vi "MultiTool-Track-Generate-ndipolarisFileOutput-Q-vectors-Standalone.vi"() -> ()   [LabVIEW 2013]
panel:
  in  "File Identifier":string="Test"
  out "TIME":string
  out "Tool 2":T1={"Port Handle"="", "Frame Number"=0, "Tx"=0.0, "Ty"=0.0, "Tz"=0.0, "Q0"=0.0, "Qx"=0.0, "Qy"=0.0, "Qz"=0.0, "Deviation"=0.0, " Markers Missing"=TRUE, "Out of Volume"=TRUE} {"Deviation" format="%#.4f"; "Qz" format="%#.4f"; "Qy" format="%#.4f"; "Qx" format="%#.4f"; "Q0" format="%#.4f"; "Tz" format="%#.2f"; "Ty" format="%#.2f"; "Tx" format="%#.2f"}
  in  "Location of ROM File for Tool 2":path=path "C:/Program Files (x86)/Northern Digital Inc/8700339.rom"
  in  "NDI  Running":bool=TRUE
  out "Stop Reading":bool=TRUE
  out "Start Reading":bool
  in  "Track Outside Measurement Volume? (F:No)":bool
  in  "Track Stray Markers? (F:No)":bool
  out "Tool 1":T1={"Port Handle"="", "Frame Number"=0, "Tx"=0.0, "Ty"=0.0, "Tz"=0.0, "Q0"=0.0, "Qx"=0.0, "Qy"=0.0, "Qz"=0.0, "Deviation"=0.0, " Markers Missing"=TRUE, "Out of Volume"=TRUE} {"Deviation" format="%#.4f"; "Qz" format="%#.4f"; "Qy" format="%#.4f"; "Qx" format="%#.4f"; "Q0" format="%#.4f"; "Tz" format="%#.2f"; "Ty" format="%#.2f"; "Tx" format="%#.2f"}
  out "Measure loop":i32
  in  "Measuring":bool=TRUE
  in  "Output Directory":path=path "C:/Users/Diogo/Desktop/NDI-Labview Gripper"
  out "NDI Loop":i32
  in  "VISA resource name":refnum<visa-resource-name>="COM8"
  in  "Reset? (T:Yes)":bool=TRUE
  in  "Location of ROM File for Tool 1":path=path "C:/Program Files (x86)/Northern Digital Inc/8700449.rom"
  in  "Serial Configuration":T2={"Baud Rate (9600)"=9600, "Flow Control (0:None)"=0, "Parity"=0, "Data Bits"=8, "Stop Bits"=10} {"Stop Bits" items=["1.0"=10, "2.0"=20]; "Parity" items=["None", "Odd", "Even"]; "Flow Control (0:None)" items=["None", "XON/XOFF"]; "Baud Rate (9600)" items=["9600"=9600, "14.4k"=14400, "19.2k"=19200, "38.4k"=38400, "57.6k "=57600, "115.2k"=115200]}
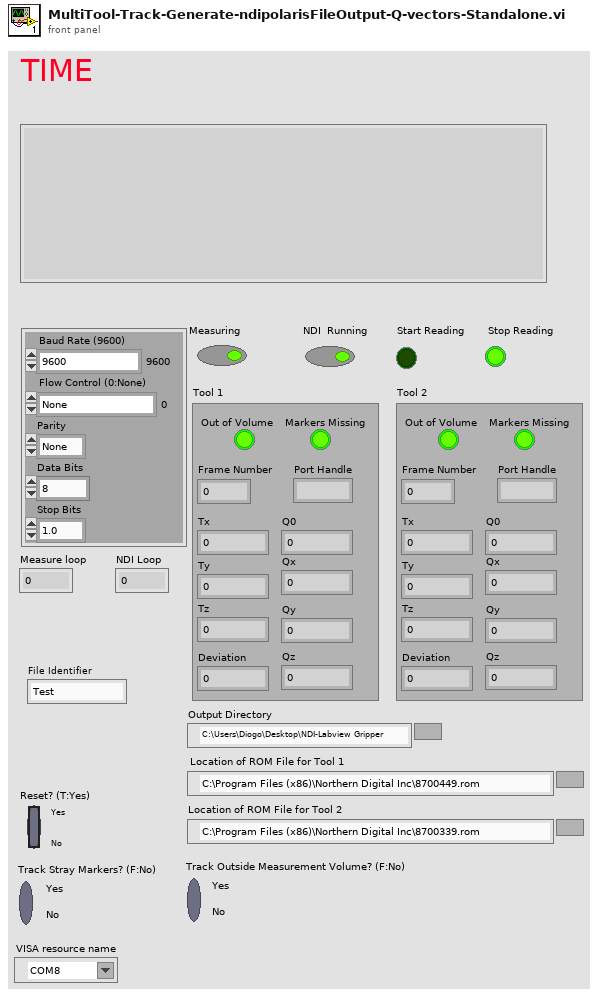
[diagram p1: front panel]
types:
  T1 = cluster{"Port Handle":string, "Frame Number":i32, "Tx":dbl, "Ty":dbl, "Tz":dbl, "Q0":dbl, "Qx":dbl, "Qy":dbl, "Qz":dbl, "Deviation":dbl, " Markers Missing":bool, "Out of Volume":bool}
  T2 = cluster{"Baud Rate (9600)":u32, "Flow Control (0:None)":u16, "Parity":u16, "Data Bits":u16, "Stop Bits":u16}
  T3 = cluster{"Port Handle":string, "Frame Number":u32, "Tx":dbl, "Ty":dbl, "Tz":dbl, "Q0":dbl, "Qx":dbl, "Qy":dbl, "Qz":dbl, "Deviation":dbl, "Missing?":bool, "Out of Volume?":bool}[]
  T4 = cluster{"Transformations[0]":cluster{"Port Handle":string, "Frame Number":u32, "Tx":dbl, "Ty":dbl, "Tz":dbl, "Q0":dbl, "Qx":dbl, "Qy":dbl, "Qz":dbl, "Deviation":dbl, "Missing?":bool, "Out of Volume?":bool}, "Transformations[1]":cluster{"Port Handle":string, "Frame Number":u32, "Tx":dbl, "Ty":dbl, "Tz":dbl, "Q0":dbl, "Qx":dbl, "Qy":dbl, "Qz":dbl, "Deviation":dbl, "Missing?":bool, "Out of Volume?":bool}, "Transformations[2]":cluster{"Port Handle":string, "Frame Number":u32, "Tx":dbl, "Ty":dbl, "Tz":dbl, "Q0":dbl, "Qx":dbl, "Qy":dbl, "Qz":dbl, "Deviation":dbl, "Missing?":bool, "Out of Volume?":bool}, "Transformations[3]":cluster{"Port Handle":string, "Frame Number":u32, "Tx":dbl, "Ty":dbl, "Tz":dbl, "Q0":dbl, "Qx":dbl, "Qy":dbl, "Qz":dbl, "Deviation":dbl, "Missing?":bool, "Out of Volume?":bool}, "Transformations[4]":cluster{"Port Handle":string, "Frame Number":u32, "Tx":dbl, "Ty":dbl, "Tz":dbl, "Q0":dbl, "Qx":dbl, "Qy":dbl, "Qz":dbl, "Deviation":dbl, "Missing?":bool, "Out of Volume?":bool}, "Transformations[5]":cluster{"Port Handle":string, "Frame Number":u32, "Tx":dbl, "Ty":dbl, "Tz":dbl, "Q0":dbl, "Qx":dbl, "Qy":dbl, "Qz":dbl, "Deviation":dbl, "Missing?":bool, "Out of Volume?":bool}, "Transformations[6]":cluster{"Port Handle":string, "Frame Number":u32, "Tx":dbl, "Ty":dbl, "Tz":dbl, "Q0":dbl, "Qx":dbl, "Qy":dbl, "Qz":dbl, "Deviation":dbl, "Missing?":bool, "Out of Volume?":bool}, "Transformations[7]":cluster{"Port Handle":string, "Frame Number":u32, "Tx":dbl, "Ty":dbl, "Tz":dbl, "Q0":dbl, "Qx":dbl, "Qy":dbl, "Qz":dbl, "Deviation":dbl, "Missing?":bool, "Out of Volume?":bool}, "Transformations[8]":cluster{"Port Handle":string, "Frame Number":u32, "Tx":dbl, "Ty":dbl, "Tz":dbl, "Q0":dbl, "Qx":dbl, "Qy":dbl, "Qz":dbl, "Deviation":dbl, "Missing?":bool, "Out of Volume?":bool}}
  T5 = cluster{"Port Handle":string, "Frame Number":u32, "Tx":dbl, "Ty":dbl, "Tz":dbl, "Q0":dbl, "Qx":dbl, "Qy":dbl, "Qz":dbl, "Deviation":dbl, "Missing?":bool, "Out of Volume?":bool}
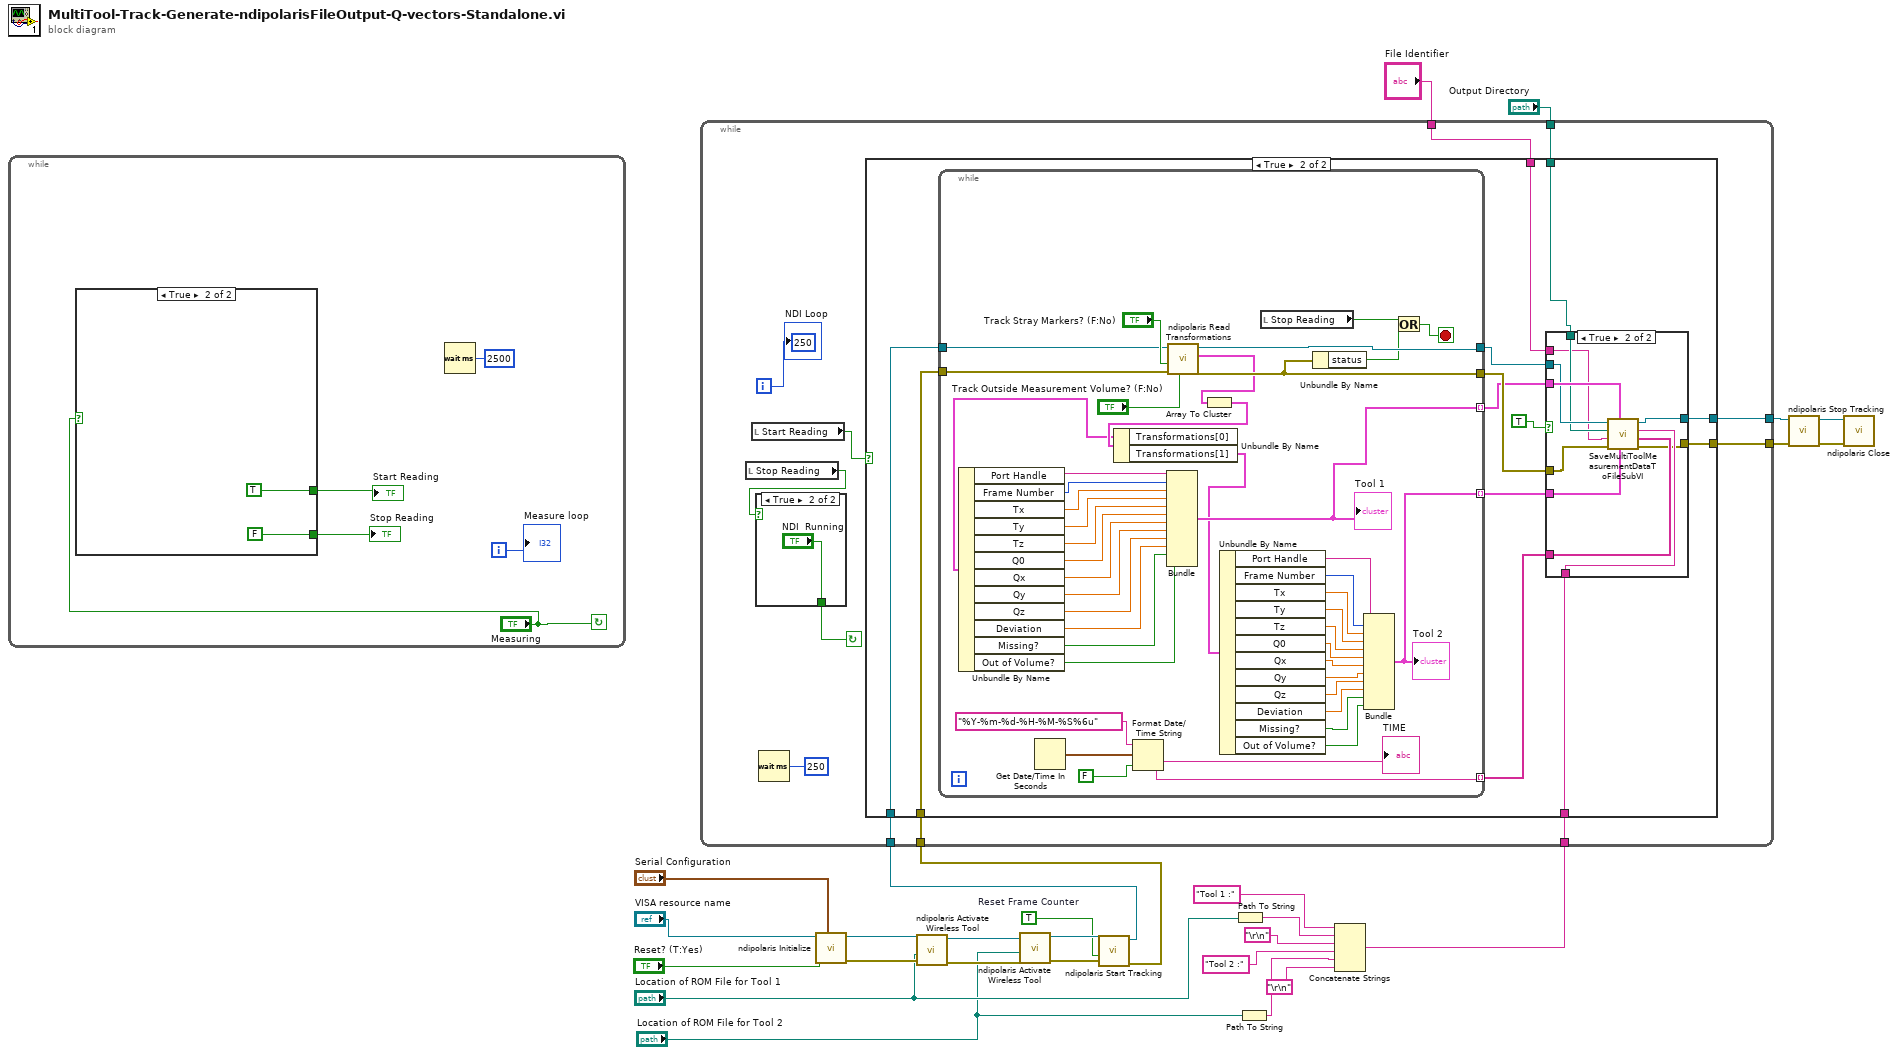
[diagram p0: block diagram]
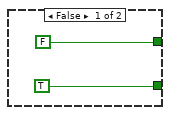
[diagram p2: hidden frame]
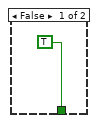
[diagram p3: hidden frame]
diagram:
  w22 = TRUE  # Reset Frame Counter
  n1 = while {
    i -> [w32]
    stop <- "Measuring" continue-if-true
    n2 = case shown="True" "Measuring" {
      tunnel: [FALSE TRUE] -> w31
      tunnel: [TRUE FALSE] -> w30
      frame False {
      }
      frame True {
      }
    }
    "Start Reading" <- w31
    "Stop Reading" <- w30
    n3 = Wait (ms)(milliseconds to wait=u32 2500) -> ()  [unwired: 1 out]
    "Measure loop" <- w32
  }
  n4 = call <instrlib>:"ndipolaris Initialize.vi"("Serial Configuration"="Serial Configuration", "Reset? (T: Yes)"="Reset? (T:Yes)", "VISA resource name"="VISA resource name") -> ("error out"=w12:errorcluster, "VISA resource name out"=w13:refnum<visa-resource-name>)  [unwired: 7 in]
  n5 = call <instrlib>:"ndipolaris Activate Wireless Tool.vi"("error in (no error)"=w12, "Location of ROM File for Tool"="Location of ROM File for Tool 1", "VISA resource name"=w13) -> ("error out"=w10:errorcluster, "VISA resource out"=w11:refnum<visa-resource-name>)  [unwired: 6 in, 1 out]
  n6 = call <instrlib>:"ndipolaris Activate Wireless Tool.vi"("error in (no error)"=w10, "Location of ROM File for Tool"="Location of ROM File for Tool 2", "VISA resource name"=w11) -> ("error out"=w23:errorcluster, "VISA resource out"=w24:refnum<visa-resource-name>)  [unwired: 6 in, 1 out]
  n7 = call <instrlib>:"ndipolaris Start Tracking.vi"("error in (no error)"=w23, "Reset Frame Counter? (F:No)"=w22, "VISA resource name"=w24) -> ("error out"=w17:errorcluster, "VISA resource out"=w21:refnum<visa-resource-name>)  [unwired: 7 in]
  n8 = Path To String(path="Location of ROM File for Tool 1") -> (string=w6:string)
  n9 = Path To String(path="Location of ROM File for Tool 2") -> (string=w4:string)
  n10 = Concatenate Strings("Tool 1 :" ("string"), w6, "\r\n", "Tool 2 :" ("string"), w4, "\r\n") -> (w14:string)
  n11 = while {
    tunnel: w21 -> [w47]
    tunnel: [w46] -> w18
    tunnel: w17 -> [w45]
    tunnel: "Output Directory" -> [w44]
    tunnel: [w43] -> w15
    tunnel: w14 -> [w38]
    tunnel: "File Identifier" -> [w37]
    i -> [w48]
    stop <- w40 continue-if-true
    (unwired) u8 250
    n12 = local read "Stop Reading"() -> (w39:bool)
    n13 = local read "Start Reading"() -> (w41:bool)
    n14 = case shown="True" w39 {
      tunnel: [TRUE "NDI  Running"] -> w40
      frame False {
      }
      frame True {
      }
    }
    n15 = Wait (ms)(milliseconds to wait=u32 250) -> ()  [unwired: 1 out]
    n16 = case shown="True" w41 {
      tunnel: w47 -> [w52 w65]
      tunnel: [w52 w62] -> w46
      tunnel: w45 -> [w51 w64]
      tunnel: w44 -> [_ w53]
      tunnel: [w51 w61] -> w43
      tunnel: w38 -> [_ w56]
      tunnel: w37 -> [_ w54]
      frame False {
      }
      frame True {
        n17 = while {
          tunnel: [w119] -> w58
          tunnel: [w118] -> w63
          tunnel: [w95] -> w59 mode=indexing
          tunnel: [w96] -> w60 mode=indexing
          tunnel: w65 -> [w94]
          tunnel: w64 -> [w93]
          tunnel: [w78] -> w55 mode=indexing
          stop <- w120 stop-if-true
          n18 = Get Date/Time In Seconds() -> (seconds since 1Jan1904=w99:timestamp)
          n19 = Format Date/Time String(time format string (%c)="%Y-%m-%d-%H-%M-%S%6u", seconds (now)=w99, UTC format=FALSE) -> (date/time string=w96:string)
          "TIME" <- w96
          n20 = call <instrlib>:"ndipolaris Read Transformations.vi"("Track Outside Measurement Volume? (F:No)"="Track Outside Measurement Volume? (F:No)", "error in (no error)"=w93, "Track Stray Markers? (F:No)"="Track Stray Markers? (F:No)", "VISA resource name"=w94) -> ("error out"=w118:errorcluster, "Transformations"=w103:T3, "VISA resource out"=w119:refnum<visa-resource-name>)  [unwired: 4 in, 1 out]
          n21 = Array To Cluster(array=w103) -> (cluster=w114:T4)
          n22 = Unbundle By Name(w114) -> ("Transformations[0]"=w113:T5, "Transformations[1]"=w91:T5)
          n23 = Unbundle By Name(w113) -> ("Port Handle"=w112:string, "Frame Number"=w111:u32, "Tx"=w110:dbl, "Ty"=w109:dbl, "Tz"=w108:dbl, "Q0"=w107:dbl, "Qx"=w106:dbl, "Qy"=w105:dbl, "Qz"=w104:dbl, "Deviation"=w102:dbl, "Missing?"=w101:bool, "Out of Volume?"=w100:bool)
          n24 = Bundle("Port Handle"=w112, "Frame Number"=w111, "Tx"=w110, "Ty"=w109, "Tz"=w108, "Q0"=w107, "Qx"=w106, "Qy"=w105, "Qz"=w104, "Deviation"=w102, "Missing?"=w101, "Out of Volume?"=w100) -> (w95:T5)  [unwired: 1 in]
          "Tool 1" <- w95
          n25 = Unbundle By Name(w91) -> ("Port Handle"=w90:string, "Frame Number"=w89:u32, "Tx"=w88:dbl, "Ty"=w87:dbl, "Tz"=w86:dbl, "Q0"=w85:dbl, "Qx"=w84:dbl, "Qy"=w83:dbl, "Qz"=w82:dbl, "Deviation"=w81:dbl, "Missing?"=w80:bool, "Out of Volume?"=w79:bool)
          n26 = local read "Stop Reading"() -> (w92:bool)
          n27 = Unbundle By Name(w118) -> ("status"=w117:bool)
          n28 = Bundle("Port Handle"=w90, "Frame Number"=w89, "Tx"=w88, "Ty"=w87, "Tz"=w86, "Q0"=w85, "Qx"=w84, "Qy"=w83, "Qz"=w82, "Deviation"=w81, "Missing?"=w80, "Out of Volume?"=w79) -> (w78:T5)  [unwired: 1 in]
          "Tool 2" <- w78
          n29 = Or(x=w92, y=w117) -> (x .or. y?=w120:bool)
        }
        n30 = case shown="True" TRUE {
          tunnel: w53 -> [_ w75]
          tunnel: w63 -> [w66 w74]
          tunnel: [w67 w73] -> w62
          tunnel: [w66 w69] -> w61
          tunnel: w60 -> [_ w72]
          tunnel: w59 -> [_ w77]
          tunnel: w58 -> [w67 w76]
          tunnel: w56 -> [_ w71]
          tunnel: w55 -> [_ w70]
          tunnel: w54 -> [_ w68]
          frame False {
          }
          frame True {
            n31 = call "SaveMultiToolMeasurementDataToFileSubVI.vi"("Array of Time for Measurement"=w72, "NDI Tool"=w71, "Array - Transformations of Tool 2"=w70, "Array - Transformations of Tool 1"=w77, "error in (no error)"=w74, "Object number"=w68, "Output Directory"=w75, "VISA Refnum in"=w76) -> ("error out"=w69:errorcluster, "VISA Refnum out"=w73:refnum<visa-resource-name>)
          }
        }
      }
    }
    "NDI Loop" <- w48
  }
  n32 = call <instrlib>:"ndipolaris Stop Tracking.vi"("error in (no error)"=w15, "VISA resource name"=w18) -> ("error out"=w19:errorcluster, "VISA resource out"=w20:refnum<visa-resource-name>)  [unwired: 8 in]
  n33 = call <instrlib>:"ndipolaris Close.vi"("error in (no error)"=w19, "VISA resource name"=w20) -> ()  [unwired: 9 in, 1 out]
